vi "Write 2D Array of String To XL.vi"(8 "error in":errorcluster, 9 "Write/Read Cell":T1={"Cell Range"="", "Data 2D"=[], "Select Sheet"="", "1 Data"="", "Data 1D"=[], "Font col"=0, "Bold"=TRUE, "Font Size"=18, "Inside lines"=FALSE}, 11 "Work Sheet":refnum<k7>) -> (0 "error out":errorcluster, 3 "Work Sheet":refnum<k7>)   [LabVIEW 2017]
uses:
  controls/read.write.ctl
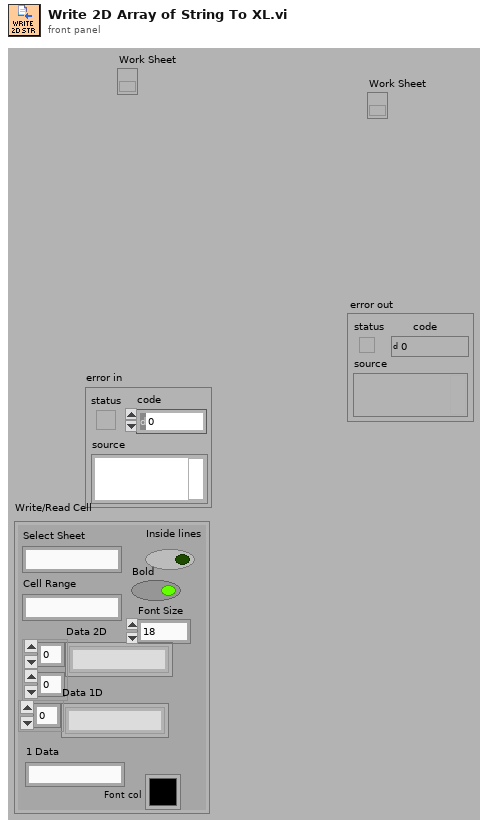
[diagram p1: front panel]
types:
  T1 = typedef "read.write.ctl" = cluster{"Cell Range":string, "Data 2D":string[][], "Select Sheet":string, "1 Data":string, "Data 1D":string[], "Font col":u32, "Bold":bool, "Font Size":i32, "Inside lines":bool}
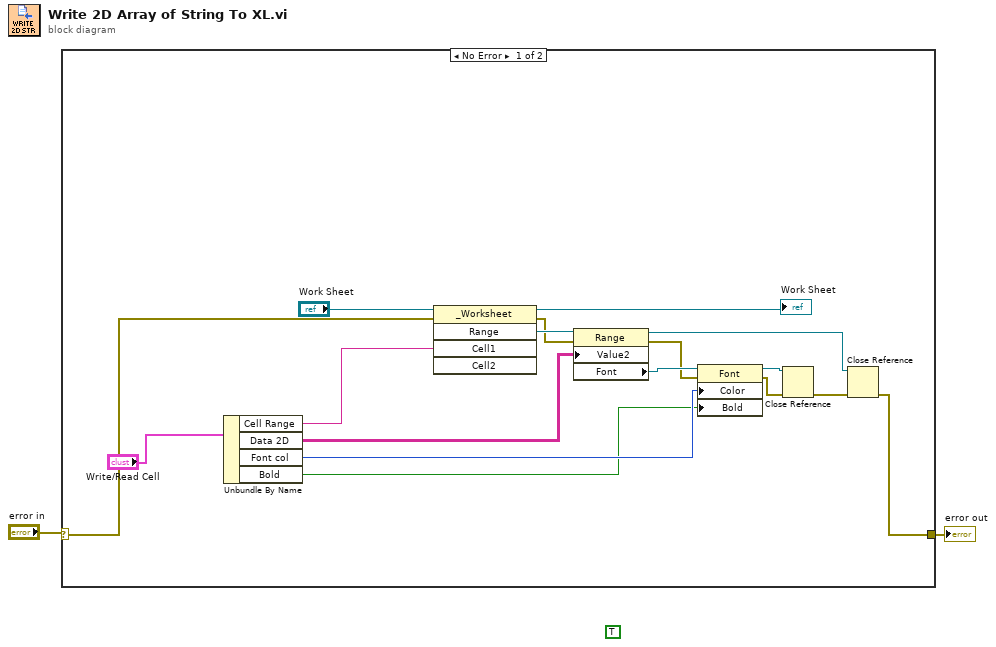
[diagram p0: block diagram]
diagram:
  (unwired) TRUE
  n1 = case shown="No Error" "error in" {
    selector: "error in" -> [w19 w20]
    tunnel: [w7 w20] -> w1
    frame No Error {
      n2 = Unbundle By Name("Write/Read Cell") -> ("Cell Range"=w4:string, "Data 2D"=w17:string[][], "Font col"=w12:u32, "Bold"=w3:bool)
      n3 = invoke class="_Worksheet" method="Range"(reference="Work Sheet", error in=w19, "Cell1"=w4) -> (reference out=→"Work Sheet":refnum<k7>, error out=w14:errorcluster, "Range"=w15:refnum<k7>)  [unwired: 2 in, 2 out]
      n4 = property class="Range"(reference=w15, error in=w14, "Value2"=w17) -> (reference out=w11:refnum<k7>, error out=w8:errorcluster, "Font"=w13:refnum<k7>)
      n5 = property class="Font"(reference=w13, error in=w8, "Color"=w12, "Bold"=w3) -> (reference out=w6:refnum<k7>, error out=w9:errorcluster)
      n6 = Close Reference(reference=w6, error in (no error)=w9) -> (error out=w10:errorcluster)
      n7 = Close Reference(reference=w11, error in (no error)=w10) -> (error out=w7:errorcluster)
    }
    frame Error {
    }
  }
  "error out" <- w1
